vi "MainMenu.vi"() -> ()   [LabVIEW 2014]
panel:
  in  "Play Tone8":bool
  in  "Tone8":path
  in  "Play Tone6":bool
  in  "Tone6":path
  in  "Play Tone5":bool
  in  "Tone5":path
  in  "Play Tone7":bool
  in  "Tone7":path
  in  "Play Tone4":bool
  in  "Tone 4":path
  in  "Play Tone3":bool
  in  "Tone3":path
  in  "Play Tone2":bool
  in  "Play Tone1":bool
  in  "Tone2":path
  in  "Tone1":path
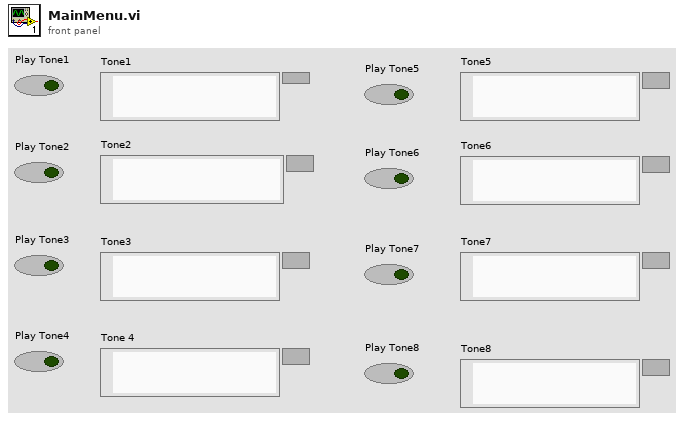
[diagram p1: front panel]
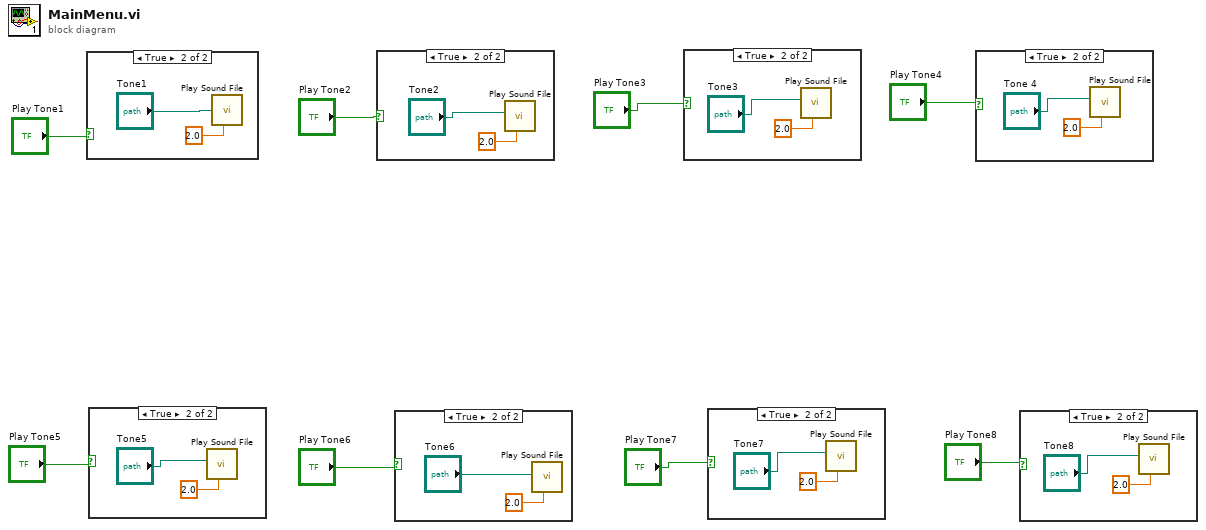
[diagram p0: block diagram]
diagram:
  n1 = case shown="True" "Play Tone1" {
    frame False {
    }
    frame True {
      n2 = call <vilib>:"Play Sound File.vi"("timeout (sec)"=2.0, "path"="Tone1") -> ()  [unwired: 8 in, 2 out]
    }
  }
  n3 = case shown="True" "Play Tone5" {
    frame False {
    }
    frame True {
      n4 = call <vilib>:"Play Sound File.vi"("timeout (sec)"=2.0, "path"="Tone5") -> ()  [unwired: 8 in, 2 out]
    }
  }
  n5 = case shown="True" "Play Tone2" {
    frame False {
    }
    frame True {
      n6 = call <vilib>:"Play Sound File.vi"("timeout (sec)"=2.0, "path"="Tone2") -> ()  [unwired: 8 in, 2 out]
    }
  }
  n7 = case shown="True" "Play Tone6" {
    frame False {
    }
    frame True {
      n8 = call <vilib>:"Play Sound File.vi"("timeout (sec)"=2.0, "path"="Tone6") -> ()  [unwired: 8 in, 2 out]
    }
  }
  n9 = case shown="True" "Play Tone3" {
    frame False {
    }
    frame True {
      n10 = call <vilib>:"Play Sound File.vi"("timeout (sec)"=2.0, "path"="Tone3") -> ()  [unwired: 8 in, 2 out]
    }
  }
  n11 = case shown="True" "Play Tone7" {
    frame False {
    }
    frame True {
      n12 = call <vilib>:"Play Sound File.vi"("timeout (sec)"=2.0, "path"="Tone7") -> ()  [unwired: 8 in, 2 out]
    }
  }
  n13 = case shown="True" "Play Tone4" {
    frame False {
    }
    frame True {
      n14 = call <vilib>:"Play Sound File.vi"("timeout (sec)"=2.0, "path"="Tone 4") -> ()  [unwired: 8 in, 2 out]
    }
  }
  n15 = case shown="True" "Play Tone8" {
    frame False {
    }
    frame True {
      n16 = call <vilib>:"Play Sound File.vi"("timeout (sec)"=2.0, "path"="Tone8") -> ()  [unwired: 8 in, 2 out]
    }
  }
